vi "FDD Algorithm Cooling OFFLINE LV2015 Ver004.vi"() -> ()   [LabVIEW 2017]
uses:
  <vilib>/Utility/file.llb/Read Delimited Spreadsheet (string).vi
  <vilib>/Utility/file.llb/Read Delimited Spreadsheet (DBL).vi
panel:
  out "Poly. Fit Coeff. HEADER Labels":string[](array[string])
  out "dT ID Air Steady 2":bool
  out "dT OD Air Steady 2":bool
  out "Cool dTsc Steady 2":bool
  out "Cooling Tsat OD Steady 2":bool
  out "Tdisch Steady 2":bool
  out "Cooling dTsh Steady 2":bool
  out "Cooling Tsat ID Steady 2":bool
  out "Data HEADER Labels":string[](array[string])
  in  "Run File?":bool
  in  "Tab Control":T1(tab)
  in  "Fault Free Polynomial's ORDER":i32=1 min=1 max=3 step=1
  out "MIN Temp":dbl
  out "MAX Temp":dbl
  out "Current Time (sec)":dbl
  in  "Time INDEX":i32=2
  in  "Tod INDEX":i32=354
  in  "Tid INDEX":i32=341
  out "Tid and Tod Drybulb-XY Graph":cluster{dbl[], dbl[]}[](graph)
  in  "Datafile Name":path=path "C:/Vance/FDD Split System Project/FY2018 Univ of Connecticut DOE FDD Project/NIST RULE BASED CHART LABVIEW FDD CODE June 2018/Example_RAW_Datafile.txt"
  out "Raw Data Array as String":string[][](array[string])
  out "Current Data Array NUMERIC-ROW":dbl[](array[numeric])
  out "HEADER Labels":string[](array[string])
  in  "Scan Pause Time (sec)":dbl=2.0 min=0.0 max=1000.0 step=0.05 format="%.2f"
  in  "Fault Free Multivariate Polynomial COEFFICIENT File Name":path=path "C:/Vance/FDD Split System Project/FY2018 Univ of Connecticut DOE FDD Project/NIST RULE BASED CHART LABVIEW FDD CODE June 2018/COEF-1st_FULL-BINNED-SS-Example_RAW_Datafile.txt"
  out "TODair, Dew Array":dbl[](array[numeric])
  out "dTDisch, sh Array":dbl[](array[numeric])
  out "Meas. COP":dbl
  in  "ID Power Index":i32=165
  out "ID Unit Power":dbl
  in  "OD Power Index":i32=168
  out "OD Unit Power":dbl
  in  "Ref. Cap Index":i32=415
  out "Cor Ref. Capacity":dbl
  in  "dT ID air St. Dev":dbl=0.5
  in  "dT OD air St. Dev":dbl=0.346
  in  "Cool dTsc St. Dev":dbl=0.8
  in  "Cooling Tsat OD St. Dev":dbl=0.5
  in  "Tdisch St. Dev":dbl=1.4
  in  "Cool dTsh St. Dev":dbl=1.0
  in  "Cooling Tsat ID St. Dev":dbl=0.6
  out "dT ID Air Steady":bool
  out "dT OD Air Steady":bool
  out "Cool dTsc Steady":bool
  out "Cooling Tsat OD Steady":bool
  out "Tdisch Steady":bool
  out "Cooling dTsh Steady":bool
  out "Cooling Tsat ID Steady":bool
  out "Cool dTsc Array":dbl[](array[numeric])
  out "Cooling Tsat ID Array":dbl[](array[numeric])
  out "Cooling Tsat OD Array":dbl[](array[numeric])
  out "Tdisch Array":dbl[](array[numeric])
  out "dT ID air Array":dbl[](array[numeric])
  out "Cool dTsh Array":dbl[](array[numeric])
  out "dT OD air Array":dbl[](array[numeric])
  out "TIDair, Dew Array":dbl[](array[numeric])
  out "TIDair, Dry Array":dbl[](array[numeric])
  out "TODair, Dry Array":dbl[](array[numeric])
  out "Meas. COP Array":dbl[](array[numeric])
  out "All Features Steady?":bool
  in  "Tidliquid":i32=401
  out "TID,liq":dbl
  in  "Todliquid":i32=383
  out "TOD,liq":dbl
  out "Cool dTsc":dbl
  out "Cool dTsh":dbl
  in  "Tdisch":i32=391
  out "Tdisch":dbl
  in  "Todairexit":i32=215
  in  "Tidairexit":i32=344
  out "TODair,exit":dbl
  out "TIDair,exit":dbl
  out "dTIDair":dbl
  out "dTODair":dbl
  in  "Tidvapor":i32=403
  out "TID,vapor":dbl
  in  "Todvapor":i32=391
  out "TOD,vapor":dbl
  out "Cooliing Tsat OD":dbl
  out "TOD,Dew":dbl
  out "TODair,Dry":dbl
  out "TIDair,Dew":dbl
  out "TIDair,Dry":dbl
  out "Cooling Tsat ID":dbl
  in  "Index Tidairdry":i32=341
  in  "Index Tidairdew":i32=242
  in  "Todairdry":i32=354
  in  "Todairdew":i32=244
  in  "Index Cool-Tsatid":i32=405
  in  "Cool-tsatod":i32=393
  out "dTdisch,sh":dbl
  in  "Moving window size":i32=10
  out "Cooling Feature StDev's":dbl[](array[numeric]) format="%_4p"
  in  "Cor RefCap":dbl
  out "Ref. Q(BTU/h)":dbl
  in  "COP COEF INDEX":i32=62
  in  "Cool dTsc COEF INDEX":i32=55
  in  "Tdisch COEF INDEX":i32=50
  in  "Cool dTsh COEF INDEX":i32=39
  in  "dT IDair COEF INDEX":i32=29
  in  "dT ODair Coef INDEX":i32=64
  in  "Cool Tsat OD Coef INDEX":i32=52
  out "Tid > Tod":bool
  in  "Cor dTsc":dbl
  in  "Cor dTsh":dbl
  in  "Cor TsatOD":dbl
  in  "COP WARNING \nPercent Degradation":dbl=-10.0
  in  "Cor dTIDair":dbl
  in  "Cor dTODair":dbl
  in  "Cor Tdisch":dbl
  in  "Cor TsatID":dbl
  out "Cooling Fault Classifier Chart":dbl[](graph) caption="Fault Classifier"
  out "Individual Probabilities (%) as Described by the RULE BASED CHART ARRAY":dbl[][](array[numeric])=[[1.0, 0.0, 1.0, -1.0, -1.0, -1.0, -1.0], [1.0, 0.0, 1.0, 1.0, -1.0, 0.0, -1.0], [-1.0, 0.0, 0.0, -1.0, 0.0, -1.0, 1.0], [-1.0, 1.0, 1.0, -1.0, 1.0, -1.0, -1.0], [0.0, 0.0, 0.0, -1.0, -1.0, -1.0, -1.0], [0.0, 0.0, 1.0, 1.0, 1.0, 0.0, 0.0], [0.0, 0.0, 0.0, 0.0, 0.0, 0.0, 0.0]] format="%.2f"
  out "Residuals":dbl[](array[numeric])=[0.583, 0.9072, 1.361, 0.43, 0.743, 0.346, 0.493]
  out "Pred. Values":dbl[](array[numeric])=[0.583, 0.9072, 1.361, 0.43, 0.743, 0.346, 0.493]
  out "Meas. Values":dbl[](array[numeric])=[0.583, 0.9072, 1.361, 0.43, 0.743, 0.346, 0.493]
  in  "Feature Thresholds":dbl[](array[numeric])=[2.56, 2.56, 2.7, 2.57, 2.57, 2.58, 2.56]
  in  "Cooling Rule Based Chart Array":dbl[][](array[numeric])=[[1.0, 0.0, 1.0, -1.0, -1.0, -1.0, -1.0], [1.0, 0.0, 1.0, 1.0, -1.0, 0.0, -1.0], [-1.0, 0.0, 0.0, -1.0, 0.0, -1.0, 1.0], [-1.0, 1.0, 1.0, -1.0, 1.0, -1.0, -1.0], [0.0, 0.0, 0.0, -1.0, -1.0, -1.0, -1.0], [0.0, 0.0, 1.0, 1.0, 1.0, 0.0, 0.0], [0.0, 0.0, 0.0, 0.0, 0.0, 0.0, 0.0]]
  out "COP % \nDegradation":dbl format="%.2g"
  out "TIDair":dbl
  out "TIDdew":dbl
  out "TODair":dbl
  out "TODdew":dbl
  out "Cool Tsat ID":dbl
  out "Cool Tsat OD":dbl
  out "dT ODair":dbl
  out "dT IDair":dbl
  out "Cool dTsh 2":dbl
  out "Tdisch 2":dbl
  out "Cool dTsc 2":dbl
  out "Avg. COP":dbl
  out "Pred. Cool Tsat ID":dbl
  out "Pred. Cool Tsat OD":dbl
  out "Pred. dT ODair":dbl
  out "Pred. dT IDair":dbl
  out "Pred. Cool dTsh":dbl
  out "Pred. Tdisch":dbl
  out "Pred. Cool dTsc":dbl
  out "Pred. COP":dbl
  out "Cooling Fault Probability":dbl[](array[numeric]) format="%_4e"
  out "EER DEGRADED?":bool
  out "Fault Occurring":bool[](array[boolean])
  out "Steady and Degraded?":bool
  in  "Cool Tsat ID Coef INDEX":i32=57
  out "Fault Occurring 2":bool[](array[boolean])
  in  "Fault #1 Row# (0 - 6)":i32=4
  out "Fault % Probabilites  - Waveform Chart 1":dbl[](graph)
  in  "NF Row# (0 - 6)":i32=6
  out "No Fault % Probabilites for Each Feature - Waveform Chart":dbl[](graph)
  out "Individual Probabilities (%) as Described by the RULE BASED CHART ARRAY 2":dbl[][](array[numeric])=[[1.0, 0.0, 1.0, -1.0, -1.0, -1.0, -1.0], [1.0, 0.0, 1.0, 1.0, -1.0, 0.0, -1.0], [-1.0, 0.0, 0.0, -1.0, 0.0, -1.0, 1.0], [-1.0, 1.0, 1.0, -1.0, 1.0, -1.0, -1.0], [0.0, 0.0, 0.0, -1.0, -1.0, -1.0, -1.0], [0.0, 0.0, 1.0, 1.0, 1.0, 0.0, 0.0], [0.0, 0.0, 0.0, 0.0, 0.0, 0.0, 0.0]] format="%.2f"
  # "FDD COOLING MODE"
  # "ALL\nSTEADY?"
  # "Index values of the same background color\nare associated with the same parameter"
  # "ROW"
  # "COL"
  # "Independent Variables"
  # "Calculated Values"
  # "Moving Window Avg. of Measured Features"
  # "Feature Steady"
  # "Cooling"
  # "Maximum Std. Deviation Allowed\nto call the feature \"STEADY\""
  # "ID Two-Phase Temp."
  # "Moving Window of Feature Values"
  # "OD Two-Phase Temp."
  # "ID vapor line"
  # "OD coil vapor inlet"
  # "Residual Values\n+1 = Positive\n-1 = Negative\n 0 = Neutral"
  # "Tsh"
  # "TD"
  # "TC"
  # "Tsc"
  # "dTCA"
  # "Te"
  # "dTEA"
  # "CMF = Comp Valve Leakage"
  # "Poly. Fit Coeff. \nINDEX (ROW#)"
  # "ODFoul = OD Coil Fouling"
  # "IDFoul = ID Coil Fouling"
  # "0.  CMF = Comp Valve Leakage"
  # "LL = Liq. Line Restriction"
  # "1.  ODFoul = OD Coil Fouling"
  # "UC = Undercharge (- %)"
  # "2.  IDFoul = ID Coil Fouling"
  # "OC = Overcharge (+ %)"
  # "3.  LL = Liq. Line Restriction"
  # "NF = No Fault"
  # "4.  UC = Undercharge (- %)"
  # "5.  OC = Overcharge (+ %)"
  # "6.  NF = No Fault"
  # "Te"
  # "Tsh"
  # "TD"
  # "TC"
  # "Tsc"
  # "dTCA"
  # "dTEA"
  # "Te"
  # "Tsh"
  # "TD"
  # "TC"
  # "Tsc"
  # "dTCA"
  # "dTEA"
  # "CMF = Comp Valve Leakage"
  # "ODFoul = OD Coil Fouling"
  # "IDFoul = ID Coil Fouling"
  # "LL = Liq. Line Restriction"
  # "UC = Undercharge (- %)"
  # "OC = Overcharge (+ %)"
  # "NF = No Fault"
  # "0.  CMF = Comp Valve Leakage"
  # "1.  ODFoul = OD Coil Fouling"
  # "2.  IDFoul = ID Coil Fouling"
  # "3.  LL = Liq. Line Restriction"
  # "4.  UC = Undercharge (- %)"
  # "5.  OC = Overcharge (+ %)"
  # "6.  NF = No Fault"
  # "Te"
  # "Tsh"
  # "TD"
  # "TC"
  # "Tsc"
  # "dTCA"
  # "dTEA"
  # "Te"
  # "Tsh"
  # "TD"
  # "TC"
  # "Tsc"
  # "dTCA"
  # "dTEA"
  # "Te"
  # "Tsh"
  # "TD"
  # "TC"
  # "Tsc"
  # "dTCA"
  # "dTEA"
  # "CMF = Comp Valve Leakage"
  # "ODFoul = OD Coil Fouling"
  # "IDFoul = ID Coil Fouling"
  # "LL = Liq. Line Restriction"
  # "UC = Undercharge (- %)"
  # "OC = Overcharge (+ %)"
  # "NF = No Fault"
  # "Feature Thresholds are determined by three types of uncertainty: 1) NF model Fit Uncertainty, 2) Measurement Uncertainty, and 3) Repeatability Uncertainty.\n\nVariances are additive.  \n\nFeature Threshold = k * sqrt( NF Model Fit Std. Error ^2 + Measurement Std. Error ^2 + Repeatability Error ^2)\nFor Example look at the included 1st order coefficient file and pull out the Mean Squared Error (MSE) for Tsat Evaporator at Row #57.  The MSE is an estimate of the fit Variance, so the square root of the MSE is the Standard Error.\n   Evap. Temp Standard Error = Tsat Evap. Temp. Error = sqrt(2.27966e-3) = 0.048 F\n   Measurement Error = 0.8 F\n   Repeatability Error = 1.0 F\n   k =2 (Greater than 95% Confidence Level on the Mean)\n\nTsat Evap or Tsat ID Threshold = 2 * sqrt((0.048)^2 + (0.8)^2 + (1.0)^2)) = 2 * 1.28 F = 2.56 F\n\nThresholds from Example File, 1st Order Fits\n           Value          Row#\nTe     = 2.56 F          57\nTsh    = 2.56            39\nTD     = 2.70            50 \nTC     = 2.57            52\nTsc    = 2.57            55 \ndTCA = 2.58            64 \ndTEA = 2.56            29"
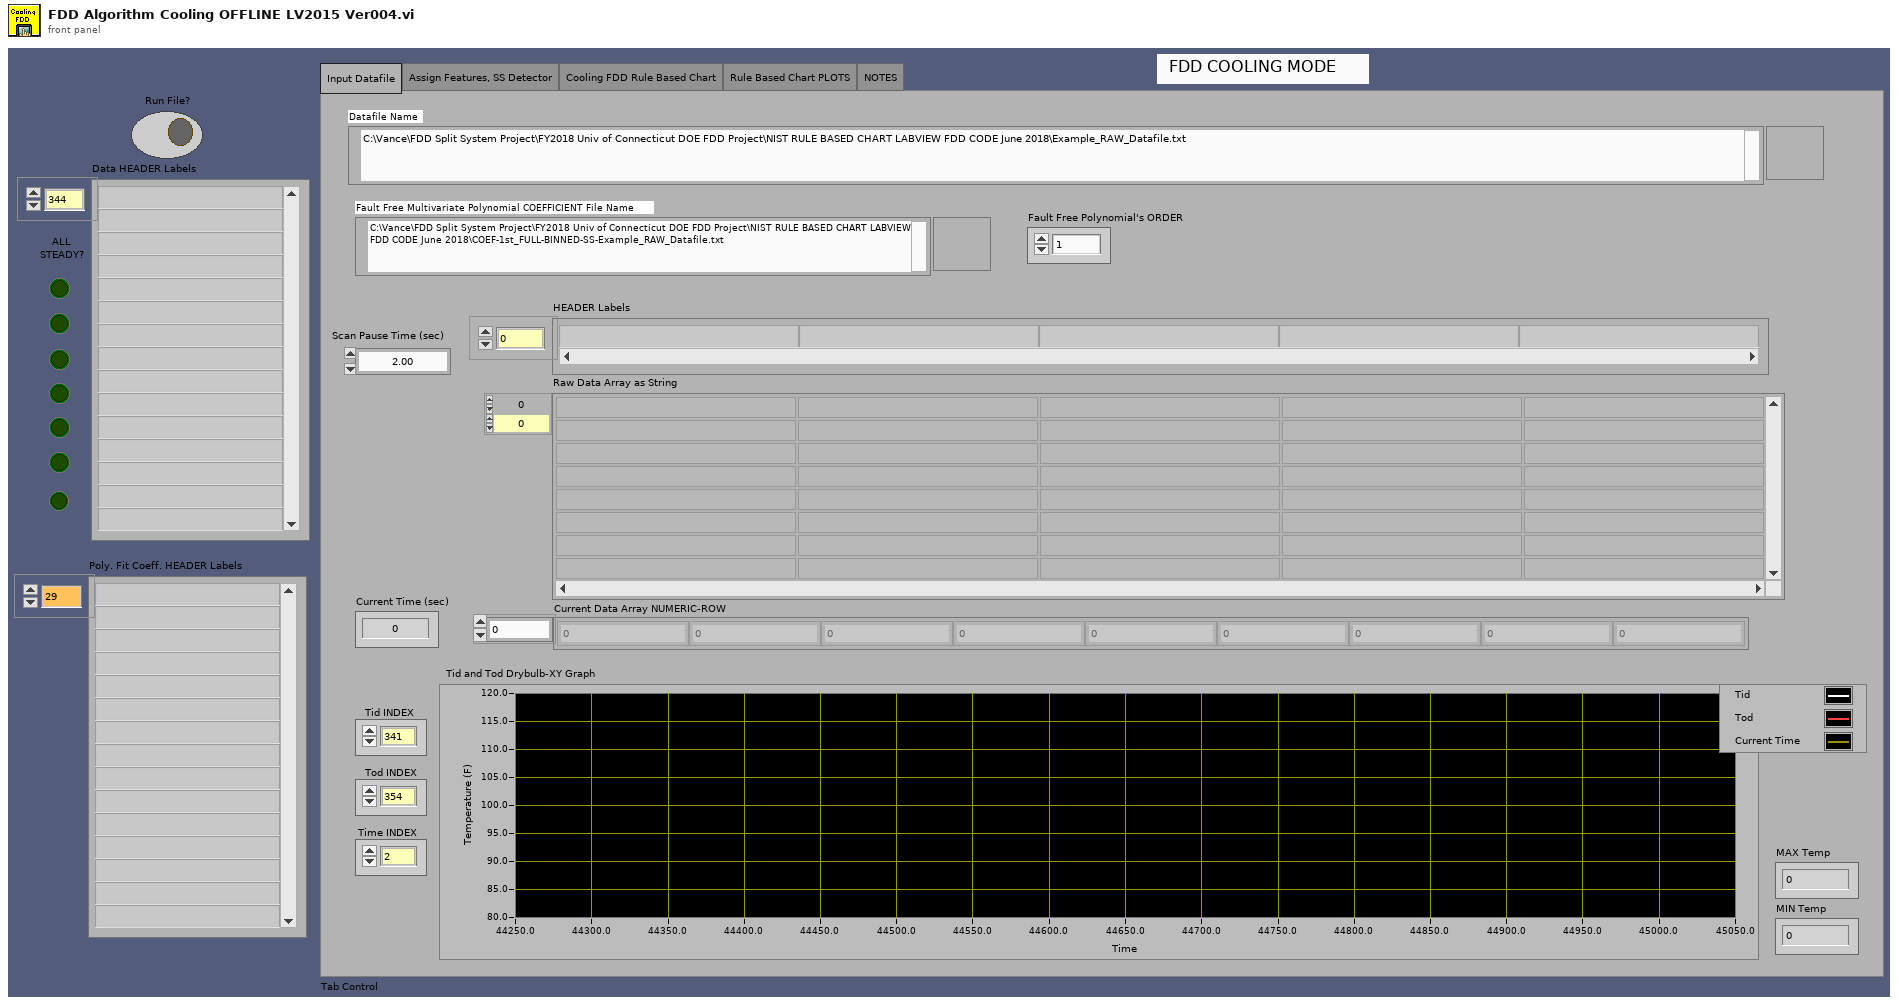
[diagram p1: front panel]
types:
  T1 = enum32{"Input Datafile", "Assign Features, SS Detector", "Cooling FDD Rule Based Chart", "Rule Based Chart PLOTS", "NOTES"}
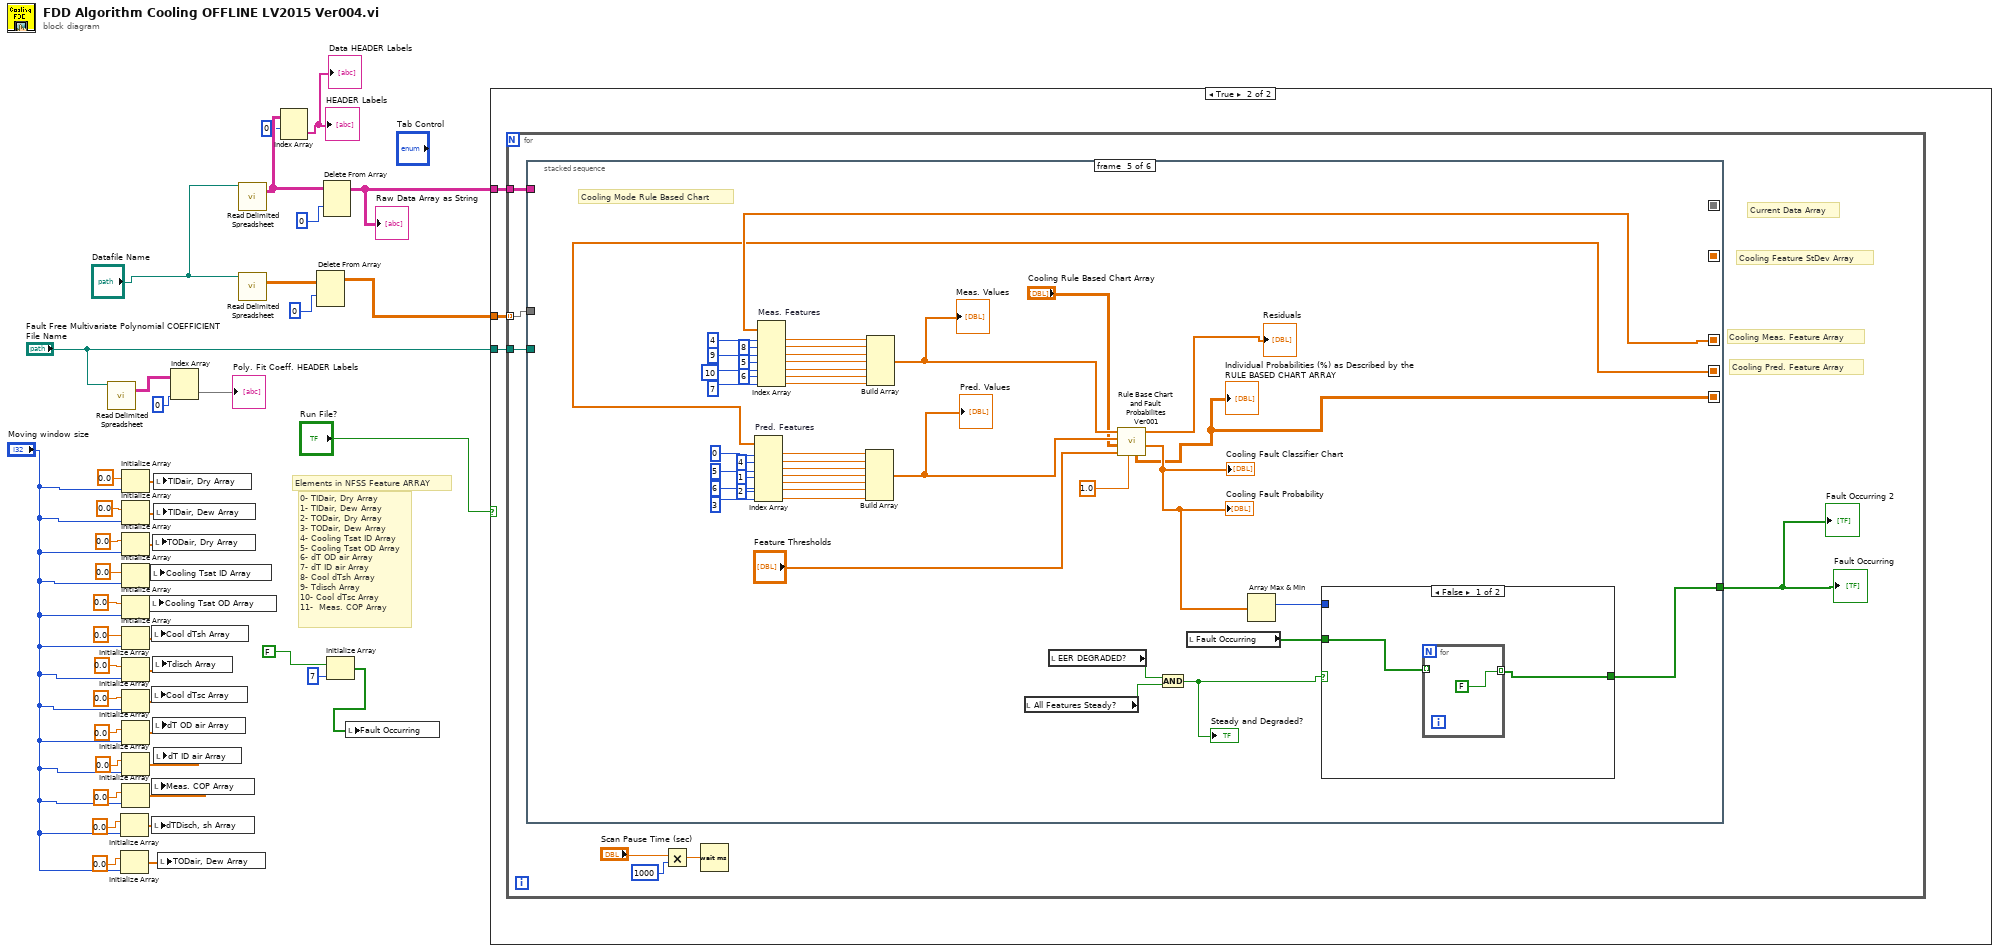
[diagram p0: block diagram]
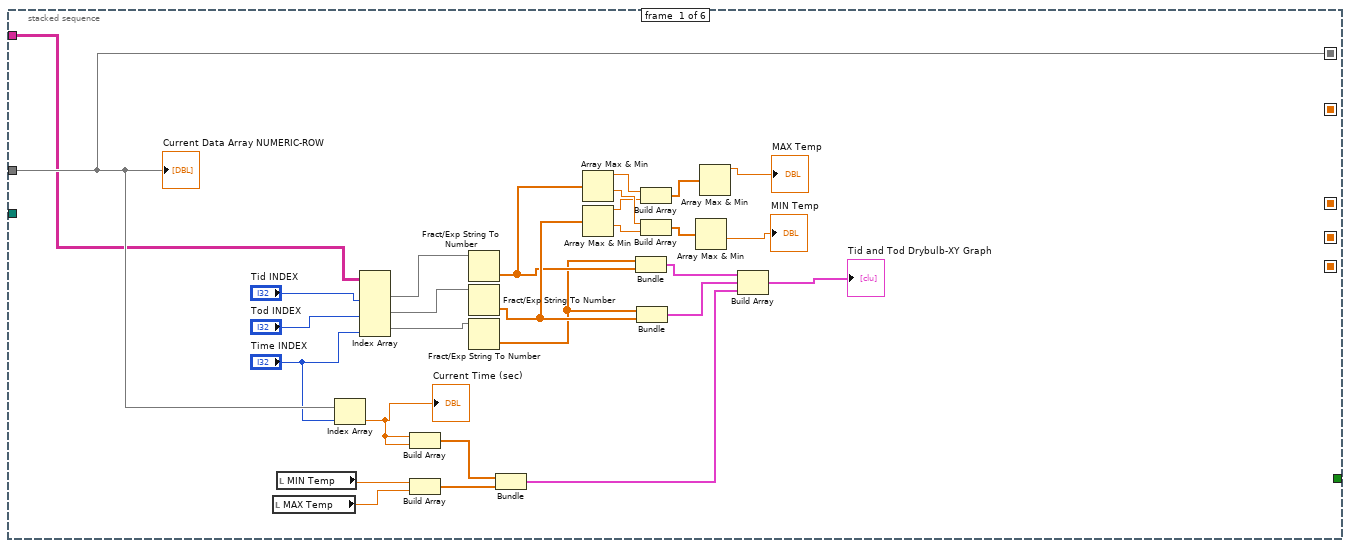
[diagram p3: hidden frame]
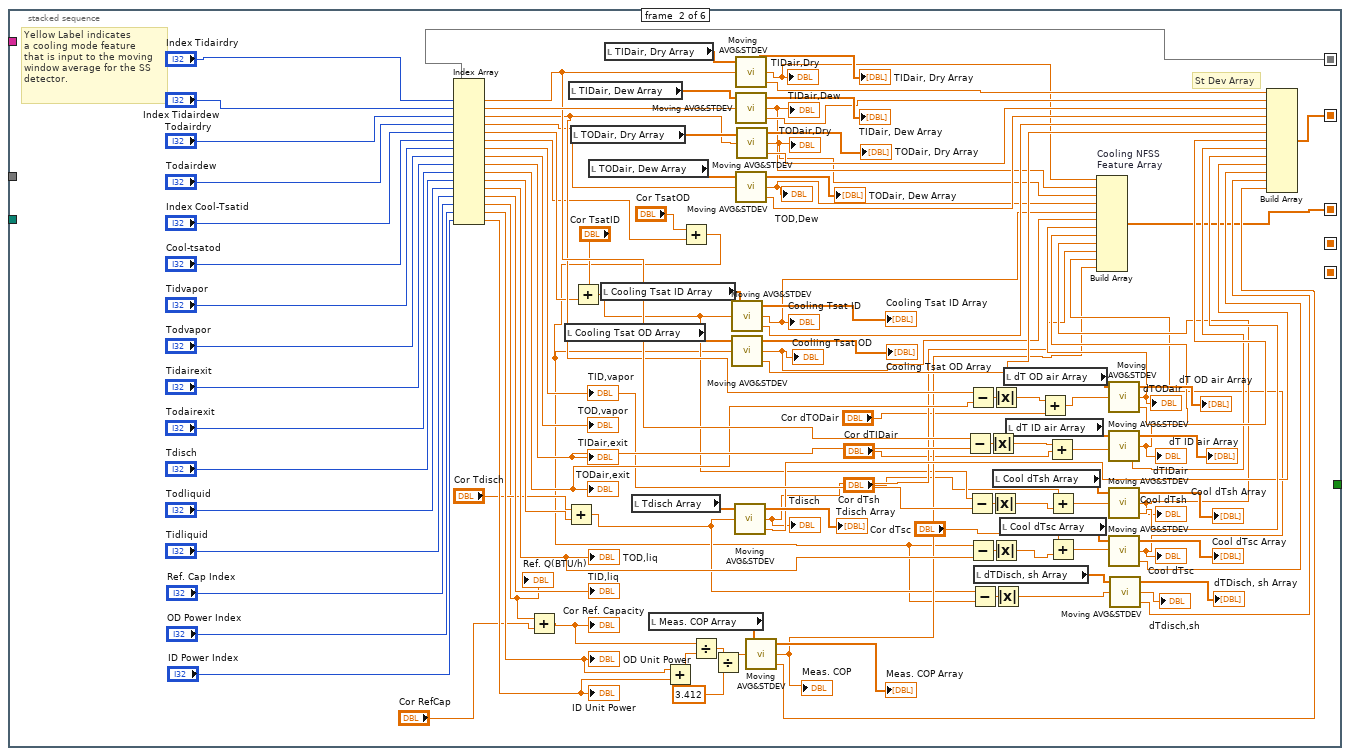
[diagram p4: hidden frame]
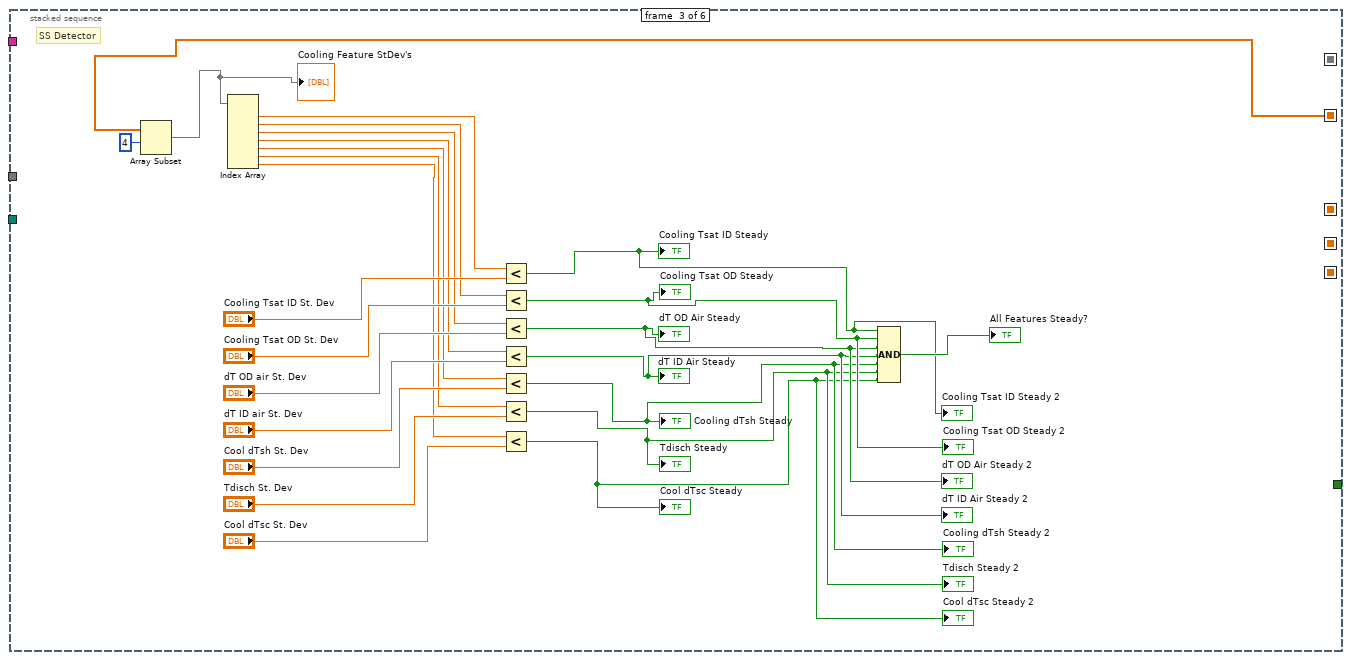
[diagram p5: hidden frame]
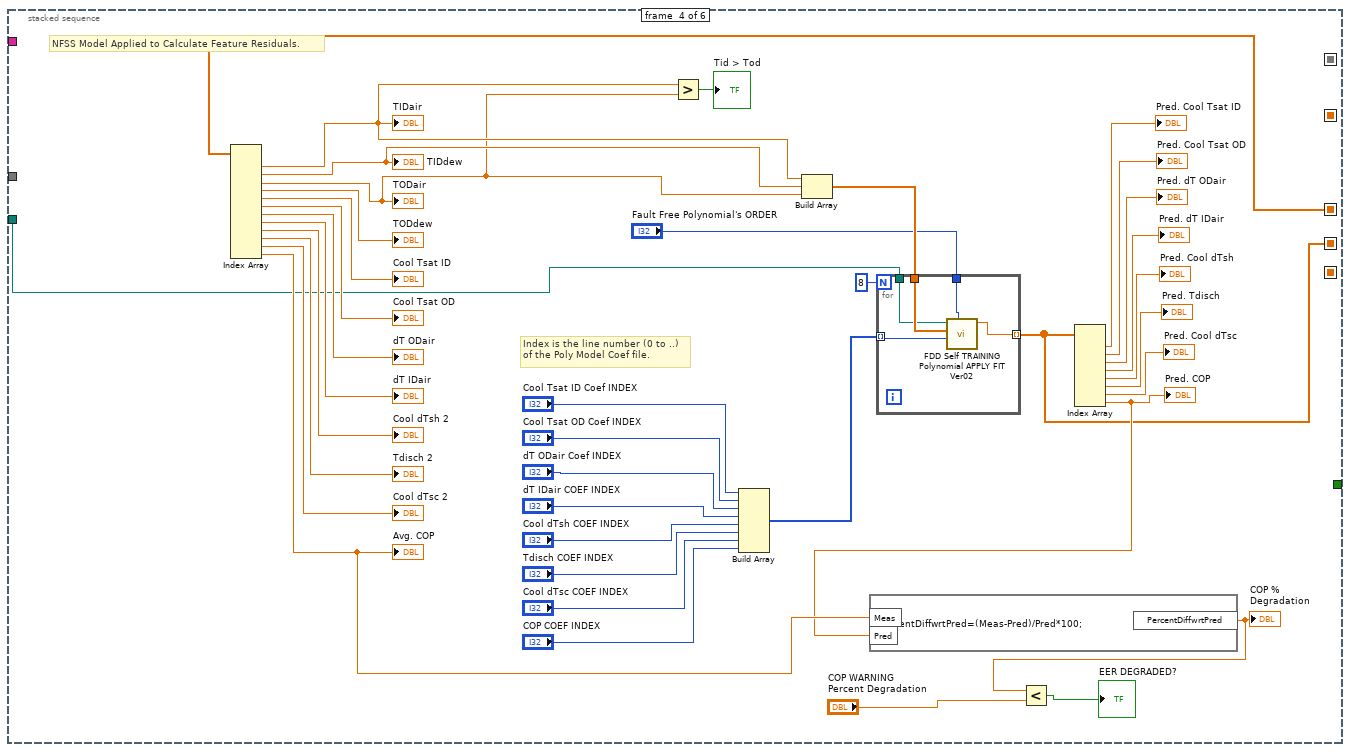
[diagram p6: hidden frame]
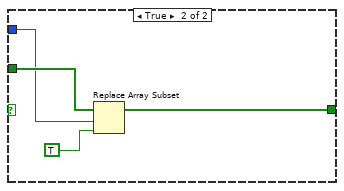
[diagram p7: hidden frame]
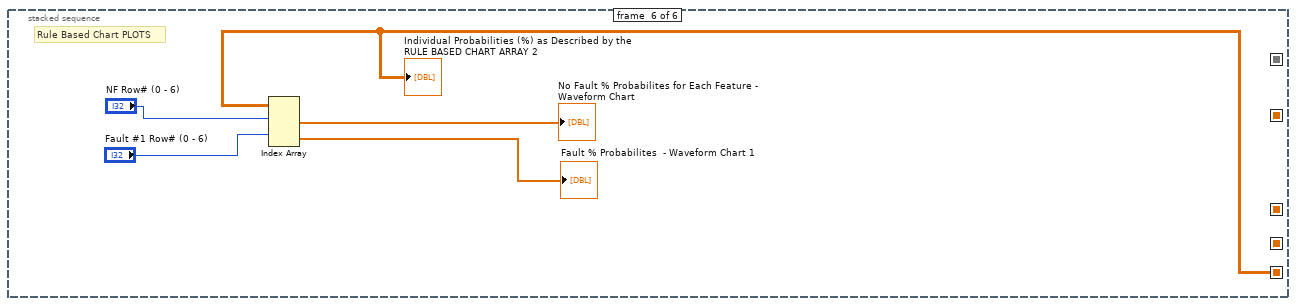
[diagram p8: hidden frame]
diagram:
  # "Elements in NFSS Feature ARRAY"
  # "0- TIDair, Dry Array\n1- TIDair, Dew Array\n2- TODair, Dry Array\n3- TODair, Dew Array\n4- Cooling Tsat ID Array\n5- Cooling Tsat OD Array\n6- dT OD air Array\n7- dT ID air Array\n8- Cool dTsh Array\n9- Tdisch Array\n10- Cool dTsc Array\n11-  Meas. COP Array"
  n1 = call-poly <vilib>:"Read Delimited Spreadsheet.vi"("file path (dialog if empty)"="Fault Free Multivariate Polynomial COEFFICIENT File Name") -> ("all rows"=w3:string[][])  [unwired: 9 in, 5 out]
  n2 = Initialize Array ("EER")(0.0 ("element"), "Moving window size") -> (w16:dbl[])
  n3 = Initialize Array ("EER")(0.0 ("element"), "Moving window size") -> (w10:dbl[])
  n4 = Initialize Array ("EER")(0.0 ("element"), "Moving window size") -> (w28:dbl[])
  n5 = Initialize Array ("EER")(0.0 ("element"), "Moving window size") -> (w27:dbl[])
  n6 = Initialize Array ("EER")(0.0 ("element"), "Moving window size") -> (w26:dbl[])
  n7 = Initialize Array ("EER")(0.0 ("element"), "Moving window size") -> (w25:dbl[])
  n8 = Initialize Array ("EER")(0.0 ("element"), "Moving window size") -> (w24:dbl[])
  n9 = Initialize Array ("EER")(0.0 ("element"), "Moving window size") -> (w23:dbl[])
  n10 = Initialize Array ("EER")(0.0 ("element"), "Moving window size") -> (w22:dbl[])
  n11 = Initialize Array ("EER")(0.0 ("element"), "Moving window size") -> (w21:dbl[])
  n12 = Initialize Array ("EER")(0.0 ("element"), "Moving window size") -> (w20:dbl[])
  n13 = Initialize Array ("EER")(0.0 ("element"), "Moving window size") -> (w19:dbl[])
  n14 = Initialize Array ("EER")(0.0 ("element"), "Moving window size") -> (w18:dbl[])
  n15 = local write "Cooling Tsat OD Array"(w24) -> ()
  n16 = local write "Cooling Tsat ID Array"(w25) -> ()
  n17 = local write "Cool dTsh Array"(w23) -> ()
  n18 = local write "Cool dTsc Array"(w21) -> ()
  n19 = local write "Meas. COP Array"(w18) -> ()
  n20 = local write "dTDisch, sh Array"(w16) -> ()
  n21 = local write "TODair, Dry Array"(w26) -> ()
  n22 = local write "Tdisch Array"(w22) -> ()
  n23 = local write "dT OD air Array"(w20) -> ()
  n24 = local write "TIDair, Dry Array"(w28) -> ()
  n25 = local write "TIDair, Dew Array"(w27) -> ()
  n26 = local write "dT ID air Array"(w19) -> ()
  n27 = local write "TODair, Dew Array"(w10) -> ()
  n28 = Index Array(array=w3, index (col)=0 ("disabled index (col)")) -> (element=→"Poly. Fit Coeff. HEADER Labels":string[])  [unwired: 1 in]
  n29 = call-poly <vilib>:"Read Delimited Spreadsheet.vi"("file path (dialog if empty)"="Datafile Name") -> ("all rows"=w9:string[][])  [unwired: 9 in, 5 out]
  n30 = call-poly <vilib>:"Read Delimited Spreadsheet.vi"("file path (dialog if empty)"="Datafile Name") -> ("all rows"=w41:dbl[][])  [unwired: 9 in, 5 out]
  n31 = Index Array(array=w9, index (row)=0) -> (element=→"HEADER Labels" →"Data HEADER Labels":string[])  [unwired: 1 in]
  n32 = Delete From Array "Delete From Array"(array=w41, index (row)=0) -> (array with subset deleted=w40:dbl[][])  [unwired: 2 in, 1 out]
  n33 = Delete From Array "Delete From Array"(array=w9, index (row)=0) -> (array with subset deleted=w5:string[][])  [unwired: 2 in, 1 out]
  "Raw Data Array as String" <- w5
  n34 = Initialize Array "Initialize Array"(FALSE, 7 ("dimension size")) -> (w13:bool[])
  n35 = local write "Fault Occurring"(w13) -> ()
  n36 = case shown="True" "Run File?" {
    tunnel: w40 -> [_ w47]
    tunnel: w5 -> [_ w46]
    tunnel: "Fault Free Multivariate Polynomial COEFFICIENT File Name" -> [_ w45]
    frame False {
    }
    frame True {
      n37 = for {
        tunnel: w47 -> [w54] mode=indexing
        tunnel: w46 -> [w49]
        tunnel: w45 -> [w48]
        # "Cooling Pred. Feature Array"
        # "Cooling Meas. Feature Array"
        # "Cooling Feature StDev Array"
        # "Current Data Array"
        n38 = stacked-sequence {
          seq-local: [w58 _ _ _ _ _] -> [_ w199 _ _ _ _]
          seq-local: [_ w123 _ _ _ _] -> [_ _ w208 _ _ _]
          seq-local: [_ w110 _ _ _ _] -> [_ _ _ w254 w311 _]
          seq-local: [_ _ _ w241 _ _] -> [_ _ _ _ w310 _]
          seq-local: [_ _ _ _ w270 _] -> [_ _ _ _ _ w324]
          tunnel: w54 -> [w58 _ _ _ _ _]
          tunnel: [_ _ _ _ w273 _] -> w50
          tunnel: w49 -> [w56 _ _ _ _ _]
          tunnel: w48 -> [_ _ _ w232 _ _]
          frame #0 {
            n39 = local read "MAX Temp"() -> (w80:dbl)
            n40 = local read "MIN Temp"() -> (w81:dbl)
            n41 = Index Array(array=w58, index="Time INDEX") -> (element=w82:dbl)
            "Current Time (sec)" <- w82
            n42 = Index Array(array=w56, index (col) #1="Tid INDEX", index (col) #2="Tod INDEX", index (col) #3="Time INDEX") -> (element #1=w61:string[], element #2=w62:string[], element #3=w63:string[])  [unwired: 3 in]
            n43 = Build Array(w82, w82) -> (w79:dbl[])
            n44 = Build Array(w81, w80) -> (w78:dbl[])
            n45 = Fract/Exp String To Number(string=w61) -> (number=w68:dbl[])  [unwired: 3 in, 1 out]
            n46 = Fract/Exp String To Number(string=w62) -> (number=w69:dbl[])  [unwired: 3 in, 1 out]
            n47 = Fract/Exp String To Number(string=w63) -> (number=w64:dbl[])  [unwired: 3 in, 1 out]
            n48 = Bundle(w79, w78) -> (w55:cluster{dbl[], dbl[]})  [unwired: 1 in]
            n49 = Array Max & Min(array=w68) -> (max value=w70:dbl, min value=w73:dbl)  [unwired: 2 out]
            n50 = Array Max & Min(array=w69) -> (max value=w71:dbl, min value=w74:dbl)  [unwired: 2 out]
            n51 = Bundle(w64, w68) -> (w65:cluster{dbl[], dbl[]})  [unwired: 1 in]
            n52 = Bundle(w64, w69) -> (w66:cluster{dbl[], dbl[]})  [unwired: 1 in]
            n53 = Build Array(w70, w71) -> (w72:dbl[])
            n54 = Build Array(w73, w74) -> (w75:dbl[])
            n55 = Array Max & Min(array=w75) -> (min value=→"MIN Temp":dbl)  [unwired: 3 out]
            n56 = Array Max & Min(array=w72) -> (max value=→"MAX Temp":dbl)  [unwired: 3 out]
            n57 = Build Array(w65, w66, w55) -> (→"Tid and Tod Drybulb-XY Graph":cluster{dbl[], dbl[]}[])
            "Current Data Array NUMERIC-ROW" <- w58
          }
          frame #1 {
            # "St Dev Array"
            # "Yellow Label indicates\na cooling mode feature\nthat is input to the moving\nwindow average for the SS \ndetector."
            n58 = Index Array(array=w199, index #1="Index Tidairdry", index #2="Index Tidairdew", index #3="Todairdry", index #4="Todairdew", index #5="Index Cool-Tsatid", index #6="Cool-tsatod", index #7="Tidvapor", index #8="Todvapor", index #9="Tidairexit", index #10="Todairexit", index #11="Tdisch", index #12="Todliquid", index #13="Tidliquid", index #14="Ref. Cap Index", index #15="OD Power Index", index #16="ID Power Index") -> (element #1=w161:dbl, element #2=w182:dbl, element #3=w155:dbl, element #4=w135:dbl, element #5=w109:dbl, element #6=w87:dbl, element #7=w151:dbl, element #8=→"TOD,vapor":dbl, element #9=w160:dbl, element #10=w154:dbl, element #11=w106:dbl, element #12=w145:dbl, element #13=→"TID,liq":dbl, element #14=w97:dbl, element #15=w167:dbl, element #16=w166:dbl)
            "TID,vapor" <- w151
            "TIDair,exit" <- w160
            "TODair,exit" <- w154
            "TOD,liq" <- w145
            "OD Unit Power" <- w167
            "ID Unit Power" <- w166
            "Ref. Q(BTU/h)" <- w97
            n59 = Add(x=w97, y="Cor RefCap") -> (x+y=w95:dbl)
            "Cor Ref. Capacity" <- w95
            n60 = local read "Cooling Tsat OD Array"() -> (w170:dbl[])
            n61 = Add(x="Cor Tdisch", y=w106) -> (x+y=w104:dbl)
            n62 = local read "TIDair, Dew Array"() -> (w180:dbl[])
            n63 = local read "TODair, Dry Array"() -> (w179:dbl[])
            n64 = Add(x="Cor TsatID", y=w109) -> (x+y=w107:dbl)
            n65 = local read "TODair, Dew Array"() -> (w134:dbl[])
            n66 = local read "Cooling Tsat ID Array"() -> (w171:dbl[])
            n67 = local read "TIDair, Dry Array"() -> (w181:dbl[])
            n68 = local read "Tdisch Array"() -> (w169:dbl[])
            n69 = local read "Meas. COP Array"() -> (w164:dbl[])
            n70 = Add(x=w167, y=w166) -> (x+y=w165:dbl)
            n71 = Add(x="Cor TsatOD", y=w87) -> (x+y=w86:dbl)
            n72 = Divide(x=w95, y=w165) -> (x/y=w85:dbl)
            n73 = Divide(x=w85, y=3.412) -> (x/y=w83:dbl)
            n74 = call "Moving AVG&STDEV.vi"("New Element for Moving Window"=w107, "Initial Array"=w171) -> ("Standard Dev"=w132:dbl, "Arithmetic Mean"=w118:dbl, "Moving Window Array"=→"Cooling Tsat ID Array":dbl[])  [unwired: 1 in]
            "Cooling Tsat ID" <- w118
            n75 = call "Moving AVG&STDEV.vi"("New Element for Moving Window"=w86, "Initial Array"=w170) -> ("Standard Dev"=w131:dbl, "Arithmetic Mean"=w117:dbl, "Moving Window Array"=→"Cooling Tsat OD Array":dbl[])  [unwired: 1 in]
            "Cooliing Tsat OD" <- w117
            n76 = call "Moving AVG&STDEV.vi"("New Element for Moving Window"=w104, "Initial Array"=w169) -> ("Standard Dev"=w125:dbl, "Arithmetic Mean"=w113:dbl, "Moving Window Array"=→"Tdisch Array":dbl[])  [unwired: 1 in]
            "Tdisch" <- w113
            n77 = call "Moving AVG&STDEV.vi"("New Element for Moving Window"=w161, "Initial Array"=w181) -> ("Standard Dev"=w139:dbl, "Arithmetic Mean"=w122:dbl, "Moving Window Array"=→"TIDair, Dry Array":dbl[])  [unwired: 1 in]
            "TIDair,Dry" <- w122
            n78 = call "Moving AVG&STDEV.vi"("New Element for Moving Window"=w182, "Initial Array"=w180) -> ("Standard Dev"=w138:dbl, "Arithmetic Mean"=w121:dbl, "Moving Window Array"=→"TIDair, Dew Array":dbl[])  [unwired: 1 in]
            "TIDair,Dew" <- w121
            n79 = call "Moving AVG&STDEV.vi"("New Element for Moving Window"=w135, "Initial Array"=w134) -> ("Standard Dev"=w133:dbl, "Arithmetic Mean"=w119:dbl, "Moving Window Array"=→"TODair, Dew Array":dbl[])  [unwired: 1 in]
            "TOD,Dew" <- w119
            n80 = call "Moving AVG&STDEV.vi"("New Element for Moving Window"=w155, "Initial Array"=w179) -> ("Standard Dev"=w137:dbl, "Arithmetic Mean"=w120:dbl, "Moving Window Array"=→"TODair, Dry Array":dbl[])  [unwired: 1 in]
            "TODair,Dry" <- w120
            n81 = call "Moving AVG&STDEV.vi"("New Element for Moving Window"=w83, "Initial Array"=w164) -> ("Standard Dev"=w124:dbl, "Arithmetic Mean"=w111:dbl, "Moving Window Array"=→"Meas. COP Array":dbl[])  [unwired: 1 in]
            "Meas. COP" <- w111
            n82 = Subtract(x=w161, y=w160) -> (x-y=w162:dbl)
            n83 = Subtract(x=w107, y=w151) -> (x-y=w152:dbl)
            n84 = Subtract(x=w155, y=w154) -> (x-y=w156:dbl)
            n85 = Subtract(x=w86, y=w145) -> (x-y=w148:dbl)
            n86 = Subtract(x=w104, y=w86) -> (x-y=w144:dbl)
            n87 = local read "dTDisch, sh Array"() -> (w140:dbl[])
            n88 = Absolute Value(x=w162) -> (abs(x)=w100:dbl)
            n89 = Absolute Value(x=w152) -> (abs(x)=w94:dbl)
            n90 = Absolute Value(x=w156) -> (abs(x)=w103:dbl)
            n91 = Absolute Value(x=w148) -> (abs(x)=w90:dbl)
            n92 = local read "Cool dTsh Array"() -> (w150:dbl[])
            n93 = Absolute Value(x=w144) -> (abs(x)=w142:dbl)
            n94 = local read "Cool dTsc Array"() -> (w146:dbl[])
            n95 = local read "dT OD air Array"() -> (w153:dbl[])
            n96 = local read "dT ID air Array"() -> (w159:dbl[])
            n97 = Add(x=w103, y="Cor dTODair") -> (x+y=w102:dbl)
            n98 = Add(x=w100, y="Cor dTIDair") -> (x+y=w99:dbl)
            n99 = Add(x="Cor dTsh", y=w94) -> (x+y=w92:dbl)
            n100 = Add(x="Cor dTsc", y=w90) -> (x+y=w91:dbl)
            n101 = call "Moving AVG&STDEV.vi"("New Element for Moving Window"=w102, "Initial Array"=w153) -> ("Standard Dev"=w130:dbl, "Arithmetic Mean"=w116:dbl, "Moving Window Array"=→"dT OD air Array":dbl[])  [unwired: 1 in]
            "dTODair" <- w116
            n102 = call "Moving AVG&STDEV.vi"("New Element for Moving Window"=w99, "Initial Array"=w159) -> ("Standard Dev"=w129:dbl, "Arithmetic Mean"=w115:dbl, "Moving Window Array"=→"dT ID air Array":dbl[])  [unwired: 1 in]
            "dTIDair" <- w115
            n103 = call "Moving AVG&STDEV.vi"("New Element for Moving Window"=w92, "Initial Array"=w150) -> ("Standard Dev"=w128:dbl, "Arithmetic Mean"=w114:dbl, "Moving Window Array"=→"Cool dTsh Array":dbl[])  [unwired: 1 in]
            "Cool dTsh" <- w114
            n104 = call "Moving AVG&STDEV.vi"("New Element for Moving Window"=w91, "Initial Array"=w146) -> ("Standard Dev"=w127:dbl, "Arithmetic Mean"=w112:dbl, "Moving Window Array"=→"Cool dTsc Array":dbl[])  [unwired: 1 in]
            "Cool dTsc" <- w112
            n105 = Build Array "Cooling NFSS\nFeature Array"(w122, w121, w120, w119, w118, w117, w116, w115, w114, w113, w112, w111) -> (w110:dbl[])
            n106 = call "Moving AVG&STDEV.vi"("New Element for Moving Window"=w142, "Initial Array"=w140) -> ("Standard Dev"=w126:dbl, "Arithmetic Mean"=→"dTdisch,sh":dbl, "Moving Window Array"=→"dTDisch, sh Array":dbl[])  [unwired: 1 in]
            n107 = Build Array(w139, w138, w137, w133, w132, w131, w130, w129, w128, w125, w127, w126, w124) -> (w123:dbl[])
          }
          frame #2 {
            # "SS Detector"
            n108 = Array Subset(array=w208, index=4) -> (w207:dbl[])  [unwired: 1 in]
            "Cooling Feature StDev's" <- w207
            n109 = Index Array(array=w207) -> (element #1=w216:dbl, element #2=w215:dbl, element #3=w214:dbl, element #4=w213:dbl, element #5=w212:dbl, element #6=w211:dbl, element #7=w210:dbl)  [unwired: 7 in]
            n110 = Less?(x=w216, y="Cooling Tsat ID St. Dev") -> (x < y?=w206:bool)
            "Cooling Tsat ID Steady" <- w206
            "Cooling Tsat ID Steady 2" <- w206
            n111 = Less?(x=w215, y="Cooling Tsat OD St. Dev") -> (x < y?=w205:bool)
            "Cooling Tsat OD Steady" <- w205
            "Cooling Tsat OD Steady 2" <- w205
            n112 = Less?(x=w214, y="dT OD air St. Dev") -> (x < y?=w204:bool)
            "dT OD Air Steady" <- w204
            "dT OD Air Steady 2" <- w204
            n113 = Less?(x=w213, y="dT ID air St. Dev") -> (x < y?=w203:bool)
            "dT ID Air Steady" <- w203
            "dT ID Air Steady 2" <- w203
            n114 = Less?(x=w212, y="Cool dTsh St. Dev") -> (x < y?=w202:bool)
            "Cooling dTsh Steady" <- w202
            "Cooling dTsh Steady 2" <- w202
            n115 = Less?(x=w211, y="Tdisch St. Dev") -> (x < y?=w201:bool)
            "Tdisch Steady" <- w201
            "Tdisch Steady 2" <- w201
            n116 = Less?(x=w210, y="Cool dTsc St. Dev") -> (x < y?=w200:bool)
            "Cool dTsc Steady" <- w200
            "Cool dTsc Steady 2" <- w200
            n117 = Compound Arithmetic op=AND(w206, w205, w204, w203, w202, w201, w200) -> (→"All Features Steady?":bool)
          }
          frame #3 {
            # "Index is the line number (0 to ..)\nof the Poly Model Coef file."
            # "NFSS Model Applied to Calculate Feature Residuals."
            n118 = Index Array(array=w254) -> (element #1=w235:dbl, element #2=w237:dbl, element #3=w234:dbl, element #4=→"TODdew":dbl, element #5=→"Cool Tsat ID":dbl, element #6=→"Cool Tsat OD":dbl, element #7=→"dT ODair":dbl, element #8=→"dT IDair":dbl, element #9=→"Cool dTsh 2":dbl, element #10=→"Tdisch 2":dbl, element #11=→"Cool dTsc 2":dbl, element #12=w243:dbl)  [unwired: 12 in]
            "TIDair" <- w235
            "TIDdew" <- w237
            "TODair" <- w234
            "Avg. COP" <- w243
            n119 = Greater?(x=w235, y=w234) -> (0:→"Tid > Tod":bool)
            n120 = Build Array("Cool Tsat ID Coef INDEX", "Cool Tsat OD Coef INDEX", "dT ODair Coef INDEX", "dT IDair COEF INDEX", "Cool dTsh COEF INDEX", "Tdisch COEF INDEX", "Cool dTsc COEF INDEX", "COP COEF INDEX") -> (w255:i32[])
            n121 = Build Array(w235, w237, w234) -> (w246:dbl[])
            n122 = for {
              N: 8 -> [_]
              tunnel: w246 -> [w268]
              tunnel: w255 -> [w266] mode=indexing
              tunnel: [w267] -> w241 mode=indexing
              tunnel: w232 -> [w265]
              tunnel: "Fault Free Polynomial's ORDER" -> [w264]
              n123 = call "FDD Self TRAINING Polynomial APPLY FIT Ver02.vi"("Polynomial ORDER\n(1st, 2nd, or 3rd)"=w264, "Which Model?\n(Row # = 0 to N)"=w266, "Independent Variables \n(3 values = Tid, Tidp, Tod)"=w268, "Coefficients with MSE File Path"=w265) -> ("Calculated or Predicted VALUE"=w267:dbl)  [unwired: 5 in, 2 out]
            }
            n124 = Index Array(array=w241) -> (element #1=→"Pred. Cool Tsat ID":dbl, element #2=→"Pred. Cool Tsat OD":dbl, element #3=→"Pred. dT ODair":dbl, element #4=→"Pred. dT IDair":dbl, element #5=→"Pred. Cool dTsh":dbl, element #6=→"Pred. Tdisch":dbl, element #7=→"Pred. Cool dTsc":dbl, element #8=w242:dbl)  [unwired: 8 in]
            "Pred. COP" <- w242
            n125 = formula code="PercentDiffwrtPred=(Meas-Pred)/Pred*100;"("Meas"=w243, "Pred"=w242) -> ("PercentDiffwrtPred"=w240:dbl)
            "COP % \nDegradation" <- w240
            n126 = Less?(x=w240, y="COP WARNING \nPercent Degradation") -> (x < y?=→"EER DEGRADED?":bool)
          }
          frame #4 {
            # "Cooling Mode Rule Based Chart"
            n127 = Index Array "Pred. Features"(array=w310, index #1=0 ("index"), index #2=4 ("index"), index #3=5 ("index"), index #4=1 ("index"), index #5=6 ("index"), index #6=2 ("index"), index #7=3 ("index")) -> (element #1=w297:dbl, element #2=w298:dbl, element #3=w299:dbl, element #4=w300:dbl, element #5=w301:dbl, element #6=w302:dbl, element #7=w303:dbl)
            n128 = Index Array "Meas. Features"(array=w311, index #1=4 ("index"), index #2=8 ("index"), index #3=9 ("index"), index #4=5 ("index"), index #5=10 ("index"), index #6=6 ("index"), index #7=7 ("index")) -> (element #1=w304:dbl, element #2=w305:dbl, element #3=w306:dbl, element #4=w307:dbl, element #5=w308:dbl, element #6=w309:dbl, element #7=w312:dbl)
            n129 = Build Array(w297, w298, w299, w300, w301, w302, w303) -> (w281:dbl[])
            "Pred. Values" <- w281
            n130 = Build Array(w304, w305, w306, w307, w308, w309, w312) -> (w282:dbl[])
            "Meas. Values" <- w282
            n131 = local read "All Features Steady?"() -> (w277:bool)
            n132 = local read "EER DEGRADED?"() -> (w278:bool)
            n133 = call "Rule Base Chart and Fault Probabilites Ver001.vi"("s - value"=1.0, "Feature Thresholds"="Feature Thresholds", "Rule Array"="Cooling Rule Based Chart Array", "Predicted Values"=w281, "Measured Values"=w282) -> ("Fault Probability"=w279:dbl[], "Residuals"=→"Residuals":dbl[], "Individual Probabilities (%)"=w270:dbl[][])  [unwired: 1 in, 3 out]
            "Cooling Fault Classifier Chart" <- w279
            "Individual Probabilities (%) as Described by the RULE BASED CHART ARRAY" <- w270
            "Cooling Fault Probability" <- w279
            n134 = And(x=w278, y=w277) -> (x .and. y?=w276:bool)
            "Steady and Degraded?" <- w276
            n135 = local read "Fault Occurring"() -> (w275:bool[])
            n136 = Array Max & Min(array=w279) -> (max index (indices)=w274:i32)  [unwired: 3 out]
            n137 = case shown="False" w276 {
              tunnel: w275 -> [w314 w319]
              tunnel: w274 -> [_ w318]
              tunnel: [w313 w317] -> w273
              frame False {
                n138 = for {
                  tunnel: w314 -> [_] mode=indexing
                  tunnel: [FALSE] -> w313 mode=indexing
                }
              }
              frame True {
                n139 = Replace Array Subset(array=w319, new element=TRUE, index=w318) -> (w317:bool[])
              }
            }
          }
          frame #5 {
            # "Rule Based Chart PLOTS"
            n140 = Index Array(array=w324, index (row) #1="NF Row# (0 - 6)", index (row) #2="Fault #1 Row# (0 - 6)") -> (element #1=→"No Fault % Probabilites for Each Feature - Waveform Chart":dbl[], element #2=→"Fault % Probabilites  - Waveform Chart 1":dbl[])  [unwired: 2 in]
            "Individual Probabilities (%) as Described by the RULE BASED CHART ARRAY 2" <- w324
          }
        }
        "Fault Occurring" <- w50
        "Fault Occurring 2" <- w50
        n141 = Multiply(x="Scan Pause Time (sec)", y=1000) -> (x*y=w53:dbl)
        n142 = Wait (ms)(milliseconds to wait=w53) -> ()  [unwired: 1 out]
      }
    }
  }
